vi "S7COMM - Parse Response - Evaluate Params.vi"(8 "error in (no error)":errorcluster, 11 "S7COMM Params and Data":T3 format="0x%02x") -> (0 "error out":errorcluster, 1 "Item Count":T2 format="0x%02x", 2 "Function Code":T1=4 items=["CPU Services"=0, "Setup Communication"=240, "Read"=4, "Write"=5], 3 "S7COMM Data":T3 format="0x%02x")   [LabVIEW 2014, in "S7NetCom.lvclass"]
uses:
  S7NetCom.lvclass
  Controls/S7NetCom_HexByteArray.ctl
  Controls/S7NetCom_HexByte.ctl
  S7COMM - Function Codes--ring.ctl
  S7COMM - Response Error Code-error.vi
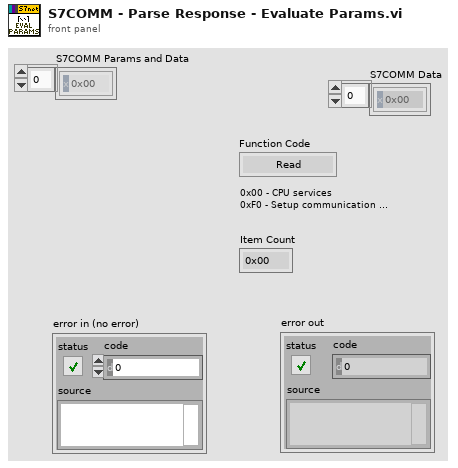
[diagram p1: front panel]
types:
  T1 = typedef "S7NetCom.lvclass/S7COMM - Function Codes--ring.ctl" = u8
  T2 = typedef "S7NetCom.lvclass/S7NetCom_HexByte.ctl" = u8
  T3 = typedef "S7NetCom.lvclass/S7NetCom_HexByteArray.ctl" = T2[]
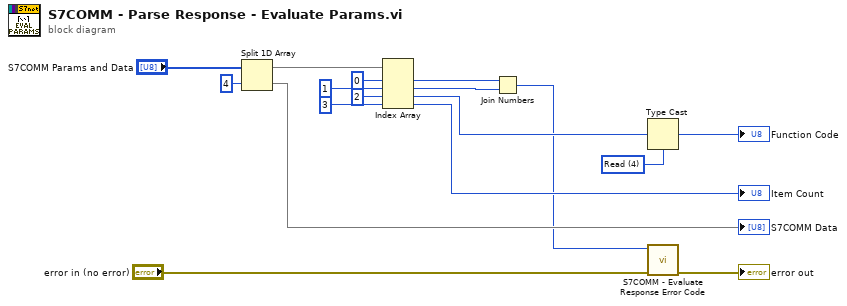
[diagram p0: block diagram]
diagram:
  w9 = T1 4 items=["CPU Services"=0, "Setup Communication"=240, "Read"=4, "Write"=5] ("Function Codes")
  n1 = Split 1D Array(array="S7COMM Params and Data", index=4) -> (first subarray=w5:T3, second subarray=→"S7COMM Data":T3)
  n2 = Index Array(array=w5, index #1=0, index #2=1, index #3=2, index #4=3) -> (element #1=w15:T2, element #2=w14:T2, element #3=w10:T2, element #4=→"Item Count":T2)
  n3 = Join Numbers(hi=w15, lo=w14) -> ((hi.lo)=w1:u16)
  n4 = Type Cast(type=w9, x=w10) -> (*(type *) &x=→"Function Code":T1)
  n5 = call "S7COMM - Evaluate Response Error Code.vi"("error in (no error)"="error in (no error)", "Error Code"=w1) -> ("error out"=→"error out":errorcluster)  [unwired: 9 in]
